vi "AdjustPuffTimingsPi3.vi"(11 "Input Trigger Data":T3) -> (3 "Output Trigger Data":T3)   [LabVIEW 2016]
uses:
  Ctrl_Signal.ctl
  Ctrl_Signal_Map.ctl
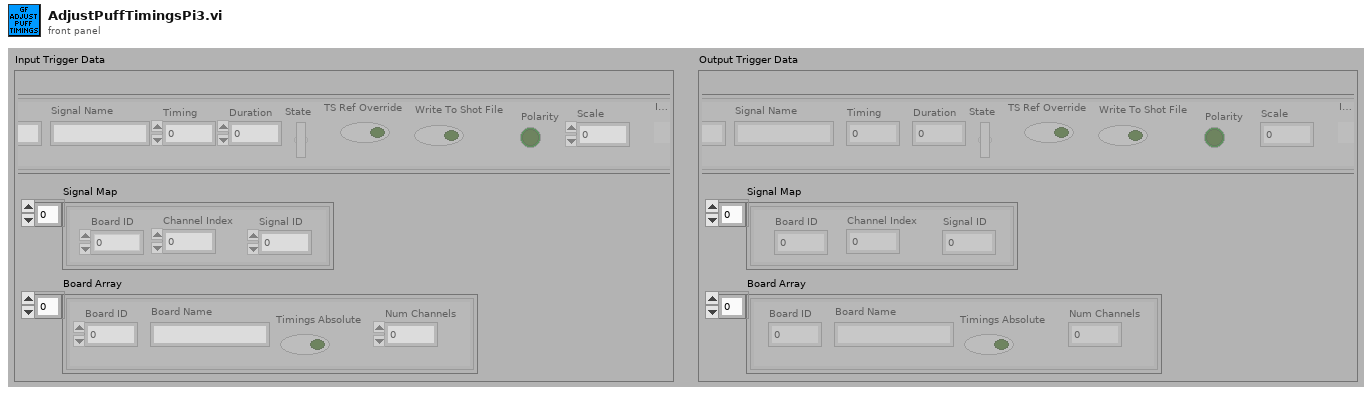
[diagram p1: front panel]
types:
  T1 = typedef "Ctrl_Signal.ctl" = cluster{"Signal Name":string, "Timing":dbl, "Duration":dbl, "State":bool, "TS Ref Override":bool, "Write To Shot File":bool, "Polarity":bool, "Signal ID":dbl, "Scale":dbl, "IsDelay":bool}
  T2 = typedef "Ctrl_Signal_Map.ctl" = cluster{"Channel Index":dbl, "Board ID":dbl, "Signal ID":dbl}
  T3 = cluster{"Signal Array":T1[], "Signal Map":T2[], "Board Array":cluster{"Board ID":dbl, "Board Name":string, "Timings Absolute":bool, "Num Channels":dbl}[]}
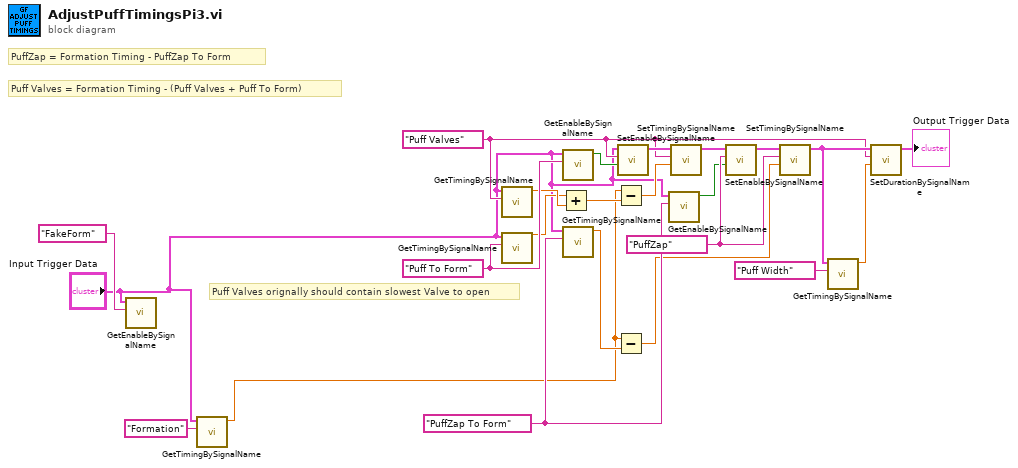
[diagram p0: block diagram]
diagram:
  w15 = "PuffZap" ("Signal Name")
  w4 = "Puff Valves" ("Signal Name")
  w22 = "PuffZap To Form" ("Signal Name")
  w21 = "Puff To Form" ("Signal Name")
  # "Puff Valves orignally should contain slowest Valve to open"
  # "PuffZap = Formation Timing - PuffZap To Form"
  # "Puff Valves = Formation Timing - (Puff Valves + Puff To Form)"
  n1 = call "GetEnableBySignalName.vi"("Signal Name"="FakeForm", "Trigger Data"="Input Trigger Data") -> ()  [unwired: 9 in, 1 out]
  n2 = call "GetTimingBySignalName.vi"("Signal Name"="Formation", "Trigger Data"="Input Trigger Data") -> ("Timing"=w1:dbl)  [unwired: 9 in]
  n3 = call "GetTimingBySignalName.vi"("Signal Name"=w4, "Trigger Data"="Input Trigger Data") -> ("Timing"=w11:dbl)  [unwired: 9 in]
  n4 = call "GetTimingBySignalName.vi"("Signal Name"=w21, "Trigger Data"="Input Trigger Data") -> ("Timing"=w10:dbl)  [unwired: 9 in]
  n5 = Add(x=w10, y=w11) -> (x+y=w9:dbl)
  n6 = call "GetEnableBySignalName.vi"("Signal Name"=w21, "Trigger Data"="Input Trigger Data") -> ("Signal Enabled"=w17:bool)  [unwired: 9 in]
  n7 = call "GetTimingBySignalName.vi"("Signal Name"=w22, "Trigger Data"="Input Trigger Data") -> ("Timing"=w13:dbl)  [unwired: 9 in]
  n8 = Subtract(x=w1, y=w9) -> (x-y=w16:dbl)
  n9 = Subtract(x=w1, y=w13) -> (x-y=w12:dbl)
  n10 = call "SetEnableBySignalName.vi"("State"=w17, "Signal Name"=w4, "Trigger Data Input"="Input Trigger Data") -> ("Trigger Data Output"=w20:T3)  [unwired: 8 in]
  n11 = call "GetEnableBySignalName.vi"("Signal Name"=w22, "Trigger Data"="Input Trigger Data") -> ("Signal Enabled"=w14:bool)  [unwired: 9 in]
  n12 = call "SetTimingBySignalName.vi"("Timing"=w16, "Signal Name"=w4, "Trigger Data Input"=w20) -> ("Trigger Data Output"=w19:T3)  [unwired: 8 in]
  n13 = call "SetEnableBySignalName.vi"("State"=w14, "Signal Name"=w15, "Trigger Data Input"=w19) -> ("Trigger Data Output"=w18:T3)  [unwired: 8 in]
  n14 = call "SetTimingBySignalName.vi"("Timing"=w12, "Signal Name"=w15, "Trigger Data Input"=w18) -> ("Trigger Data Output"=w7:T3)  [unwired: 8 in]
  n15 = call "GetTimingBySignalName.vi"("Signal Name"="Puff Width", "Trigger Data"=w7) -> ("Timing"=w5:dbl)  [unwired: 9 in]
  n16 = call "SetDurationBySignalName.vi"("Duration"=w5, "Signal Name"=w4, "Trigger Data Input"=w7) -> ("Trigger Data Output"=→"Output Trigger Data":T3)  [unwired: 8 in]
